vi "SortImageArray (SubVI).vi"(8 "error in (no error)":errorcluster, 9 "Evaluate Set of Fiducials":enum16{"mark B", "mark C"}(ring), 10 "Sequence Length":i32=8, 11 "Images Array":T1[](array[plugin-control])) -> (0 "error out":errorcluster, 2 "Sorted Images Array":T1[](array[typedef]))   [LabVIEW 2016]
uses:
  <vilib>/vision/Image Controls.llb/IMAQ Image.ctl
panel:
  out "size(s)":i32
  in  "Selected Images Subarray":T1[](array[plugin-control])
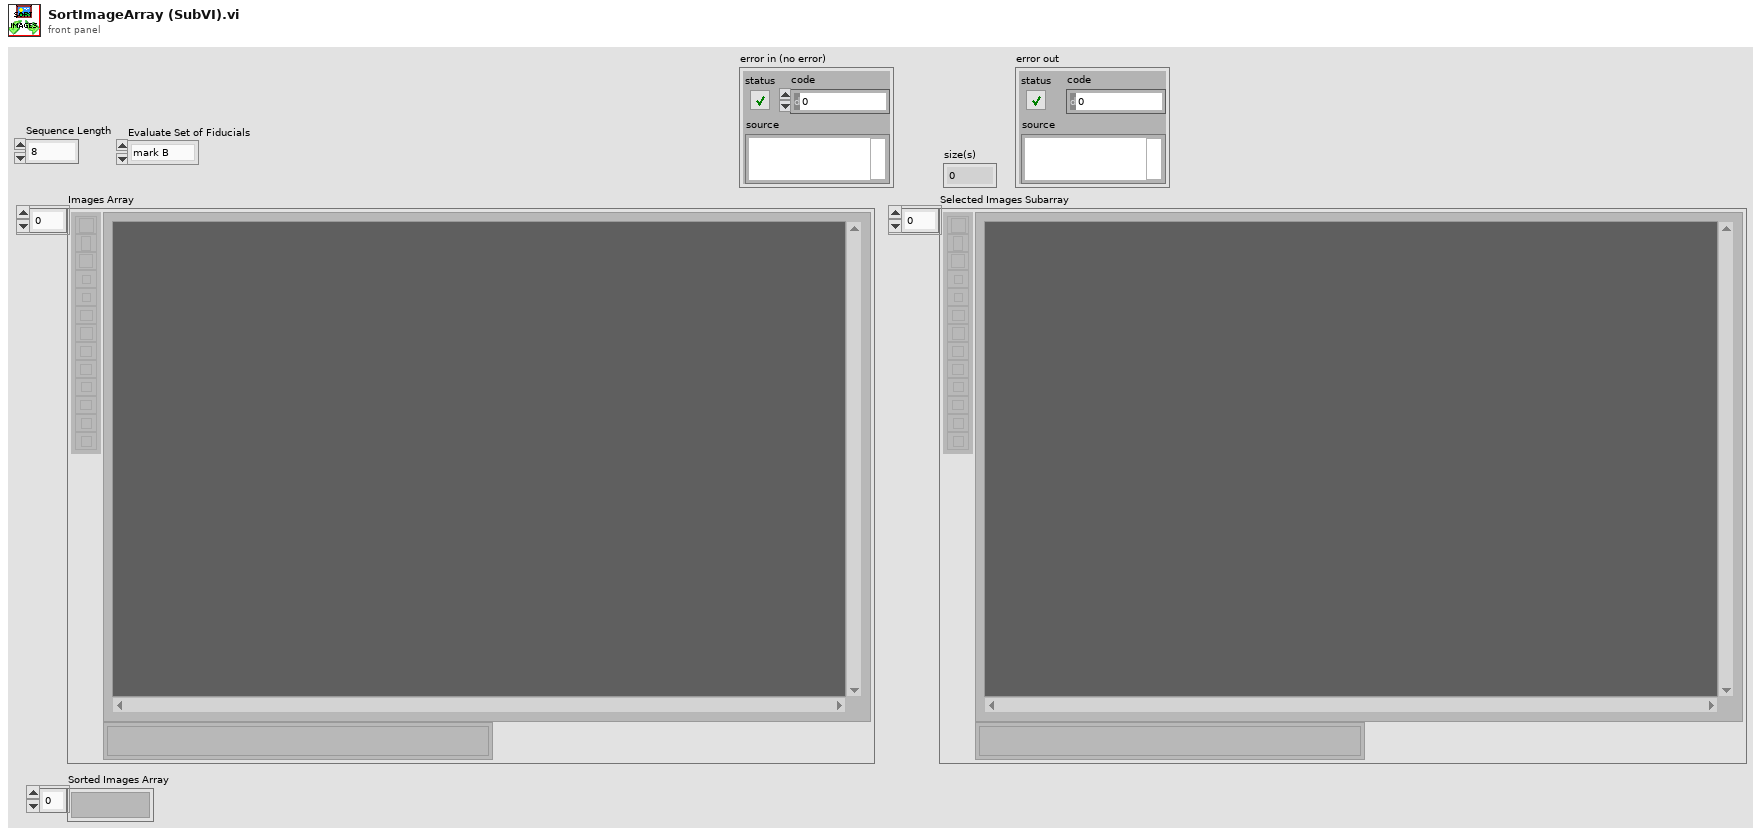
[diagram p1: front panel]
types:
  T1 = typedef "IMAQ Image.ctl" = refnum<image>
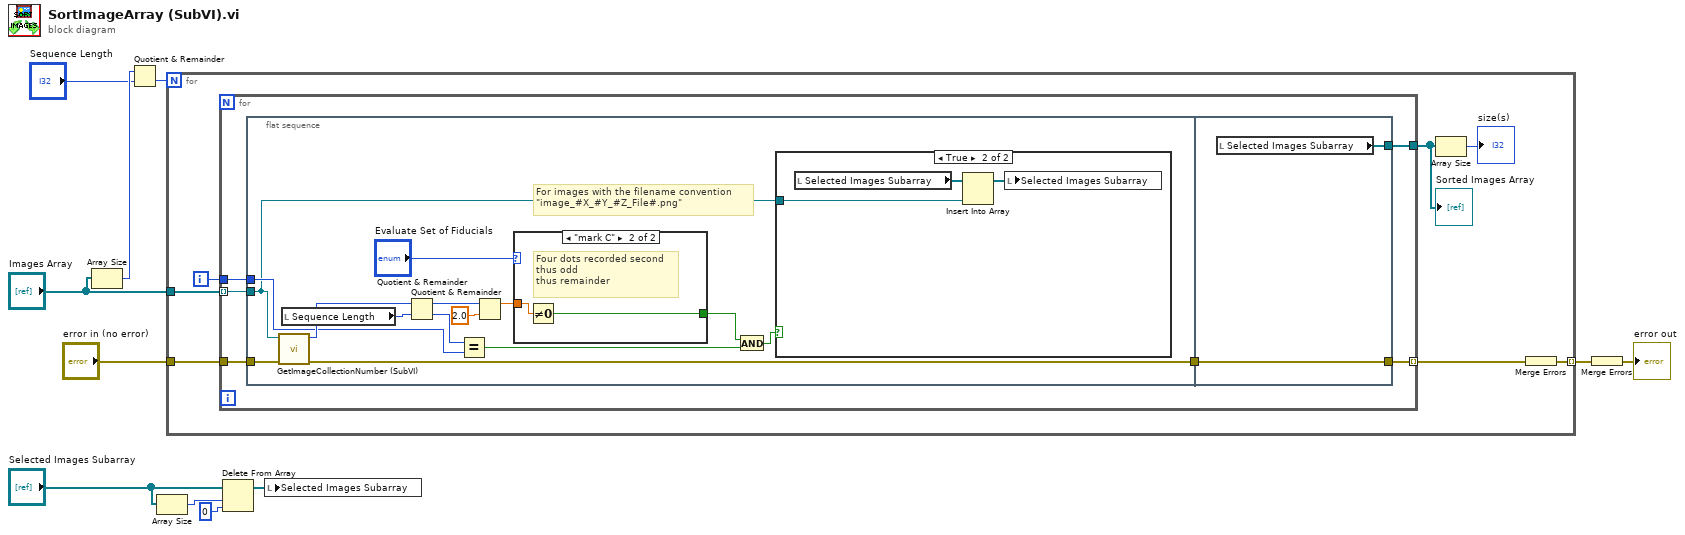
[diagram p0: block diagram]
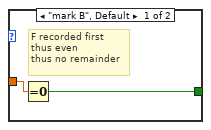
[diagram p2: hidden frame]
diagram:
  n1 = Array Size(array="Images Array") -> (size(s)=w8:i32)
  n2 = Quotient & Remainder(x=w8, y="Sequence Length") -> (floor(x/y)=w6:i32)  [unwired: 1 out]
  n3 = Array Size(array="Selected Images Subarray") -> (size(s)=w10:i32)
  n4 = for {
    N: w6 -> [_]
    tunnel: "Images Array" -> [w18]
    tunnel: "error in (no error)" -> [w15]
    tunnel: [w13] -> w2 mode=indexing
    i -> [w17]
    n5 = for {
      tunnel: w18 -> [w24] mode=indexing
      tunnel: w17 -> [w23]
      tunnel: [w22] -> w12
      tunnel: w15 -> [w21]
      tunnel: [w19] -> w14 mode=indexing
      n6 = flat-sequence {
        tunnel: w24 -> [w30]
        tunnel: w23 -> [w32]
        tunnel: w21 -> [w26]
        tunnel: [w25] -> w20
        tunnel: [w47] -> w22
        tunnel: w20 -> [w46]
        tunnel: [w46] -> w19
        frame #0 {
          # "For images with the filename convention\n\"image_#X_#Y_#Z_File#.png\""
          n7 = call "GetImageCollectionNumber (SubVI).vi"("error in (no error)"=w26, "Image in"=w30) -> ("error out"=w25:errorcluster, "Image #"=w33:i32)  [unwired: 8 in]
          n8 = local read "Sequence Length"() -> (w31:i32)
          n9 = Quotient & Remainder(x=w33, y=w31) -> (x-y*floor(x/y)=w37:i32, floor(x/y)=w38:i32)
          n10 = Equal?(x=w38, y=w32) -> (x = y?=w35:bool)
          n11 = Quotient & Remainder(x=w37, y=2.0) -> (x-y*floor(x/y)=w28:dbl)  [unwired: 1 out]
          n12 = case shown="\"mark C\"" "Evaluate Set of Fiducials" {
            tunnel: w28 -> [w40 w42]
            tunnel: [w39 w41] -> w27
            frame "mark B", Default {
              # "F recorded first\nthus even\nthus no remainder"
              n13 = Equal To 0?(x=w40) -> (x = 0?=w39:bool)
            }
            frame "mark C" {
              # "Four dots recorded second\nthus odd\nthus remainder"
              n14 = Not Equal To 0?(x=w42) -> (x != 0?=w41:bool)
            }
          }
          n15 = And(x=w27, y=w35) -> (x .and. y?=w34:bool)
          n16 = case shown="True" w34 {
            tunnel: w30 -> [_ w43]
            frame False {
            }
            frame True {
              n17 = local read "Selected Images Subarray"() -> (w45:T1[])
              n18 = Insert Into Array(array=w45, new element=w43) -> (w44:T1[])  [unwired: 1 in]
              n19 = local write "Selected Images Subarray"(w44) -> ()
            }
          }
        }
        frame #1 {
          n20 = local read "Selected Images Subarray"() -> (w47:T1[])
        }
      }
    }
    "Sorted Images Array" <- w12
    n21 = Array Size(array=w12) -> (size(s)=→"size(s)":i32)
    n22 = Merge Errors(w14) -> (w13:errorcluster)
  }
  n23 = Delete From Array(array="Selected Images Subarray", length=w10, index=0) -> (array with subset deleted=w11:T1[])  [unwired: 1 out]
  n24 = local write "Selected Images Subarray"(w11) -> ()
  n25 = Merge Errors(w2) -> (→"error out":errorcluster)
